vi "NtfyLvFpga_SUB__cutoffLine_MultiLineString.vi"(9 "LineCount at End(1000)":i32=1000 min=1, 11 "String":string) -> (3 "String out":string)   [LabVIEW 2013]
uses:
  <vilib>/Utility/error.llb/whitespace.ctl
panel:
  # "複数行文字列の末尾から指定した行数を残して、それ以外を削除する。\nログ表示などのように、大量に追加されていく文字列が長くなりすぎないように、\n最新の(末尾からの)1000行以上は削除して表示したい時などに利用する。"
  # "末尾からの行数"
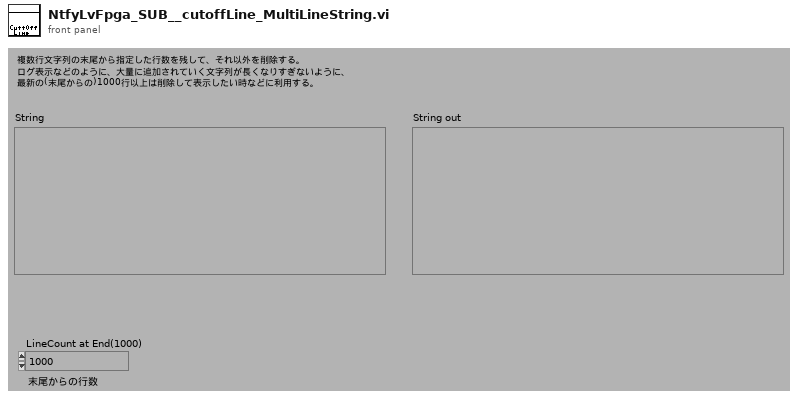
[diagram p1: front panel]
types:
  T1 = typedef "whitespace.ctl" = u16
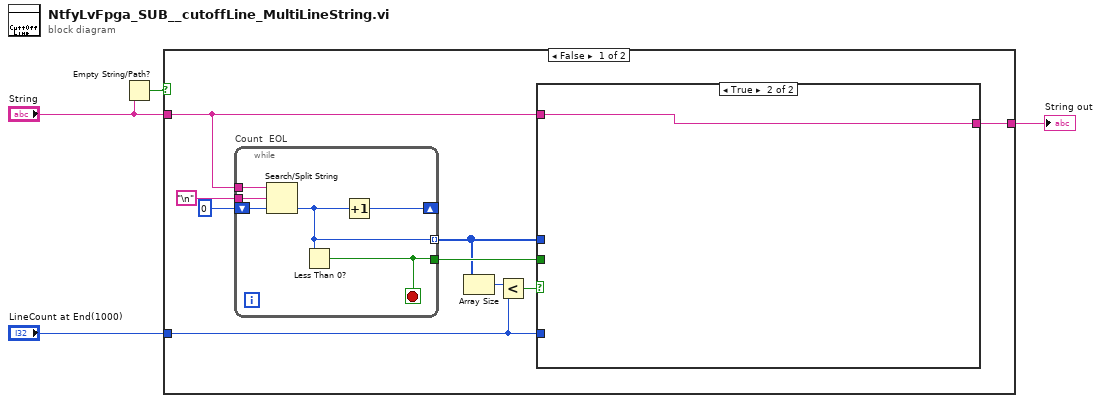
[diagram p0: block diagram]
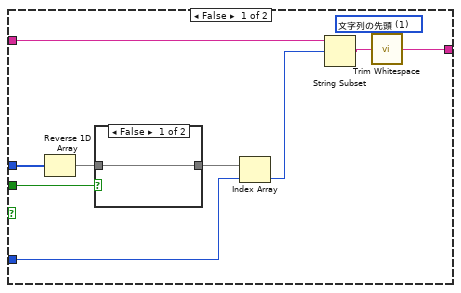
[diagram p2: hidden frame]
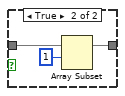
[diagram p3: hidden frame]
diagram:
  n1 = Empty String/Path?(string/path="String") -> (empty?=w2:bool)
  n2 = case shown="FALSE" w2 {
    tunnel: "LineCount at End(1000)" -> [w5 _]
    tunnel: "String" -> [w10 _]
    tunnel: [w9 _] -> w3
    frame False {
      n3 = while "Count  EOL" {
        tunnel: w10 -> [w34]
        tunnel: "\n" -> [w33]
        tunnel: [w31] -> w7 mode=indexing
        tunnel: [w32] -> w11
        shift-right: [w29] -> _
        shift-left: 0 ("offset of match") -> [w30]
        stop <- w32 stop-if-true
        n4 = Search/Split String(string=w34, search string/char (-)=w33, offset (0)=w30) -> (offset of match=w31:i32)  [unwired: 2 out]
        n5 = Less Than 0?(x=w31) -> (x < 0?=w32:bool)
        n6 = Increment(x=w31) -> (x+1=w29:i32)
      }
      n7 = Array Size(array=w7) -> (size(s)=w8:i32)
      n8 = Less?(x=w8, y=w5) -> (x < y?=w6:bool)
      n9 = case shown="TRUE" w6 {
        tunnel: w5 -> [w23 _]
        tunnel: w7 -> [w22 _]
        tunnel: w11 -> [w21 _]
        tunnel: w10 -> [w18 w28]
        tunnel: [w15 w28] -> w9
        frame False {
          w14 = T1 1 items=["両方", "文字列の先頭", "文字列の終わり"] ("location (both)")
          n10 = Reverse 1D Array(array=w22) -> (reversed array=w20:i32[])
          n11 = case shown="FALSE" w21 {
            tunnel: w20 -> [w24 w25]
            tunnel: [w24 w26] -> w19
            frame False {
            }
            frame True {
              n12 = Array Subset(array=w25, index=1 ("指標")) -> (w26:i32[])  [unwired: 1 in]
            }
          }
          n13 = Index Array(array=w19, index=w23) -> (element=w16:i32)
          n14 = String Subset(string=w18, offset (0)=w16) -> (substring=w17:string)  [unwired: 1 in]
          n15 = call <vilib>:"Trim Whitespace.vi"("string"=w17, "location (both)"=w14) -> ("trimmed string"=w15:string)
        }
        frame True {
        }
      }
    }
    frame True {
    }
  }
  "String out" <- w3
